vi "Host_Model_Updating.vi"(11 "Setup Parameters and Controls":T3={"Modeling Parameters input controls"={"beam_length"=0.3525, "youngs_modulus"=209500000000.0, "torsion_spring"=0.0, "beam_height"=0.00635, "beam_width"=0.0508, "beam_density"=7900.0, "number_of_FEA_nodes"=40, "accelerometer_mass"=0.055}, "Mockbear input controls"={"Dataset"="test7", "Resample Method"=enum."Auto Resample"}, "Simulation Parameters input controls"={"Eigensolver "=enum."LEMP", "Models Forcasted"=5, "Max Roller Velocity"=3.32, "Max Roller Position Percent"=0.43, "Min Roller Position Percent"=0.155}, "Program Controls"={"Frequency KF"=TRUE, "Pinned State KF"=FALSE, "FFT Bounding"=FALSE, "Filter Constants Frequency"={"Measurement Variance"=0.4, "State Variance"=0.01, "Threshold"=1000000000.0}, "Filter Constants Position"={"Measurement Variance"=0.4, "State Variance"=0.9, "Threshold"=1000000000.0}, "Moving Window Size"=10, "Time Series buffer"=10000.0, "Record Time Series Data"=FALSE, "Record Moving Window Data"=FALSE, "Record Online Error Metrics "=TRUE, "Record Statistics"=TRUE}}) -> ()   [LabVIEW 2021]
uses:
  Model_Updating_Classes/DROPBEAR_Model_Updating/DROPBEAR_Model_Updating.lvclass
panel:
  in  "Halt":bool
  in  "Tab Control":enum32{"Time Series", "Statistics", "Controls"}(tab)
  out "Frequency":dynamicdata(graph)
  out "Meter":dynamicdata(graph)
  out "Nodal":dynamicdata(graph)
  out "DAQ Time cost":T1
  out "FFT Time cost":T1
  out "FEA Time cost":T1
  out "FFT KF Time cost":T1
  out "Sampling Time cost":T1
  out "State KF Time cost":T1
  out "Cycle Time cost":T1
  out "StatisticsTime cost":T1
  out "Signal Quality Stats Frequency":T2
  out "Signal Quality Stats Position":T2
  out "Average Cycle Time (ms)":dbl
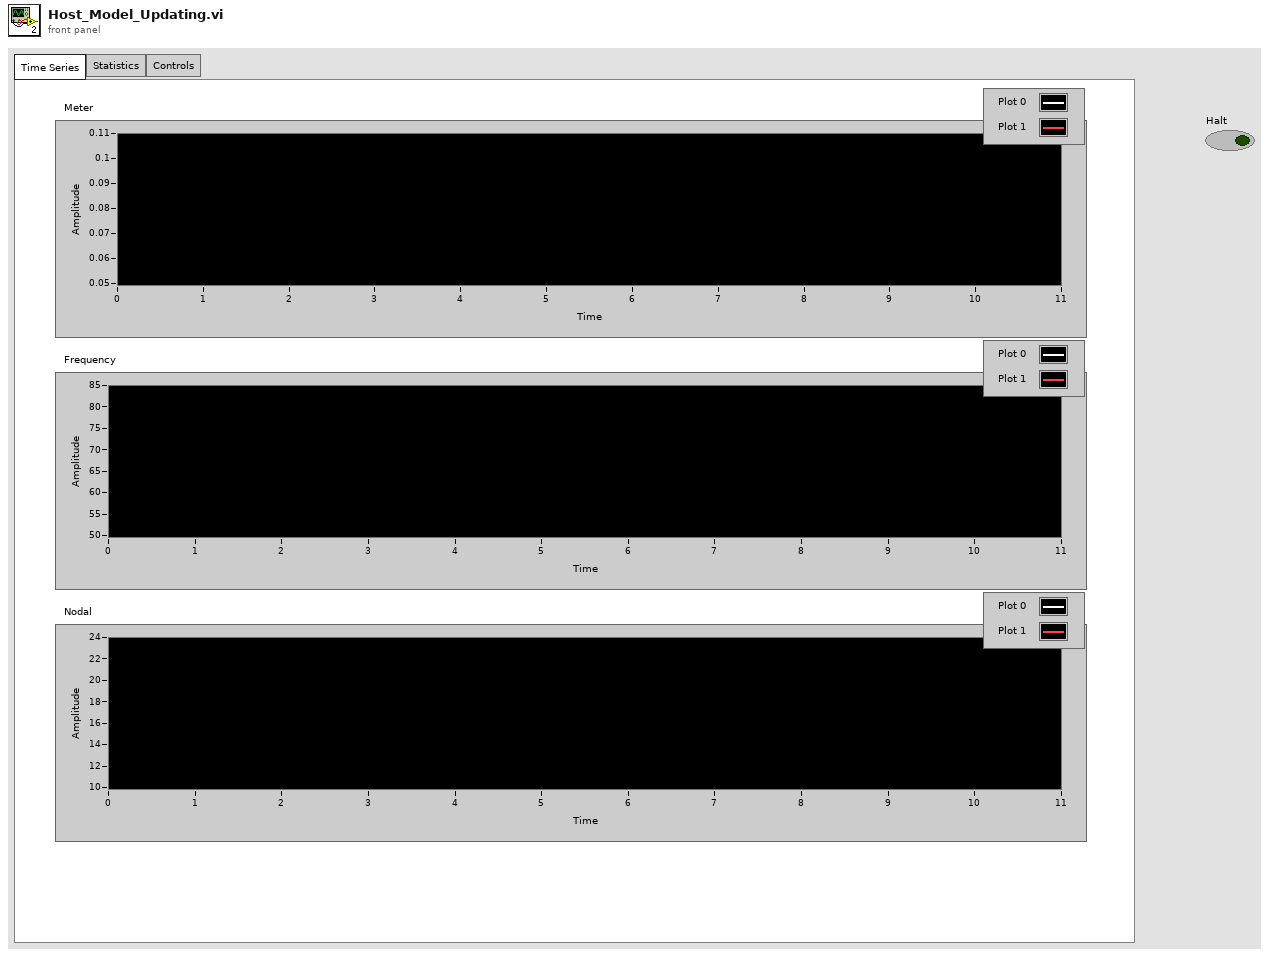
[diagram p1: front panel]
types:
  T1 = cluster{"Cumulative_mean":dbl, "Cumulative_mean_square ":dbl, "Cumulative_variance":dbl, "Max":dbl, "Min":dbl, "Number_of_samples":i32}
  T2 = cluster{"SNR":dbl, "TRAC":dbl, "Cumulative_mean":dbl, "Cumulative_mean_square ":dbl, "Cumulative_variance":dbl, "Max":dbl, "Min":dbl, "Number_of_samples":i32}
  T3 = cluster{"Modeling Parameters input controls":cluster{"beam_length":dbl, "youngs_modulus":dbl, "torsion_spring":dbl, "beam_height":dbl, "beam_width":dbl, "beam_density":dbl, "number_of_FEA_nodes":i32, "accelerometer_mass":dbl}, "Mockbear input controls":cluster{"Dataset":string, "Resample Method":enum16{"Recorded", "Auto Resample", "Custom Resample"}}, "Simulation Parameters input controls":cluster{"Eigensolver ":enum16{"LabVIEW Cholesky", "LabVIEW General", "LabVIEW Inverse", "LEMP"}, "Models Forcasted":i32, "Max Roller Velocity":dbl, "Max Roller Position Percent":dbl, "Min Roller Position Percent":dbl}, "Program Controls":cluster{"Frequency KF":bool, "Pinned State KF":bool, "FFT Bounding":bool, "Filter Constants Frequency":cluster{"Measurement Variance":dbl, "State Variance":dbl, "Threshold":dbl}, "Filter Constants Position":cluster{"Measurement Variance":dbl, "State Variance":dbl, "Threshold":dbl}, "Moving Window Size":i32, "Time Series buffer":dbl, "Record Time Series Data":bool, "Record Moving Window Data":bool, "Record Online Error Metrics ":bool, "Record Statistics":bool}}
  T4 = cluster{"Signal Quality Stats Frequency":cluster{"SNR":dbl, "TRAC":dbl, "Cumulative_mean":dbl, "Cumulative_mean_square ":dbl, "Cumulative_variance":dbl, "Max":dbl, "Min":dbl, "Number_of_samples":i32}, "Signal Quality Stats Position":cluster{"SNR":dbl, "TRAC":dbl, "Cumulative_mean":dbl, "Cumulative_mean_square ":dbl, "Cumulative_variance":dbl, "Max":dbl, "Min":dbl, "Number_of_samples":i32}}
  T5 = cluster{"DAQ Time cost":cluster{"Cumulative_mean":dbl, "Cumulative_mean_square ":dbl, "Cumulative_variance":dbl, "Max":dbl, "Min":dbl, "Number_of_samples":i32}, "FFT Time cost":cluster{"Cumulative_mean":dbl, "Cumulative_mean_square ":dbl, "Cumulative_variance":dbl, "Max":dbl, "Min":dbl, "Number_of_samples":i32}, "FFT KF Time cost":cluster{"Cumulative_mean":dbl, "Cumulative_mean_square ":dbl, "Cumulative_variance":dbl, "Max":dbl, "Min":dbl, "Number_of_samples":i32}, "Sampling Time cost":cluster{"Cumulative_mean":dbl, "Cumulative_mean_square ":dbl, "Cumulative_variance":dbl, "Max":dbl, "Min":dbl, "Number_of_samples":i32}, "FEA Time cost":cluster{"Cumulative_mean":dbl, "Cumulative_mean_square ":dbl, "Cumulative_variance":dbl, "Max":dbl, "Min":dbl, "Number_of_samples":i32}, "State KF Time cost":cluster{"Cumulative_mean":dbl, "Cumulative_mean_square ":dbl, "Cumulative_variance":dbl, "Max":dbl, "Min":dbl, "Number_of_samples":i32}, "Cycle Time cost":cluster{"Cumulative_mean":dbl, "Cumulative_mean_square ":dbl, "Cumulative_variance":dbl, "Max":dbl, "Min":dbl, "Number_of_samples":i32}, "StatisticsTime cost":cluster{"Cumulative_mean":dbl, "Cumulative_mean_square ":dbl, "Cumulative_variance":dbl, "Max":dbl, "Min":dbl, "Number_of_samples":i32}}
  T6 = cluster{"Frequency":dynamicdata, "Meters":dynamicdata, "Nodal":dynamicdata}
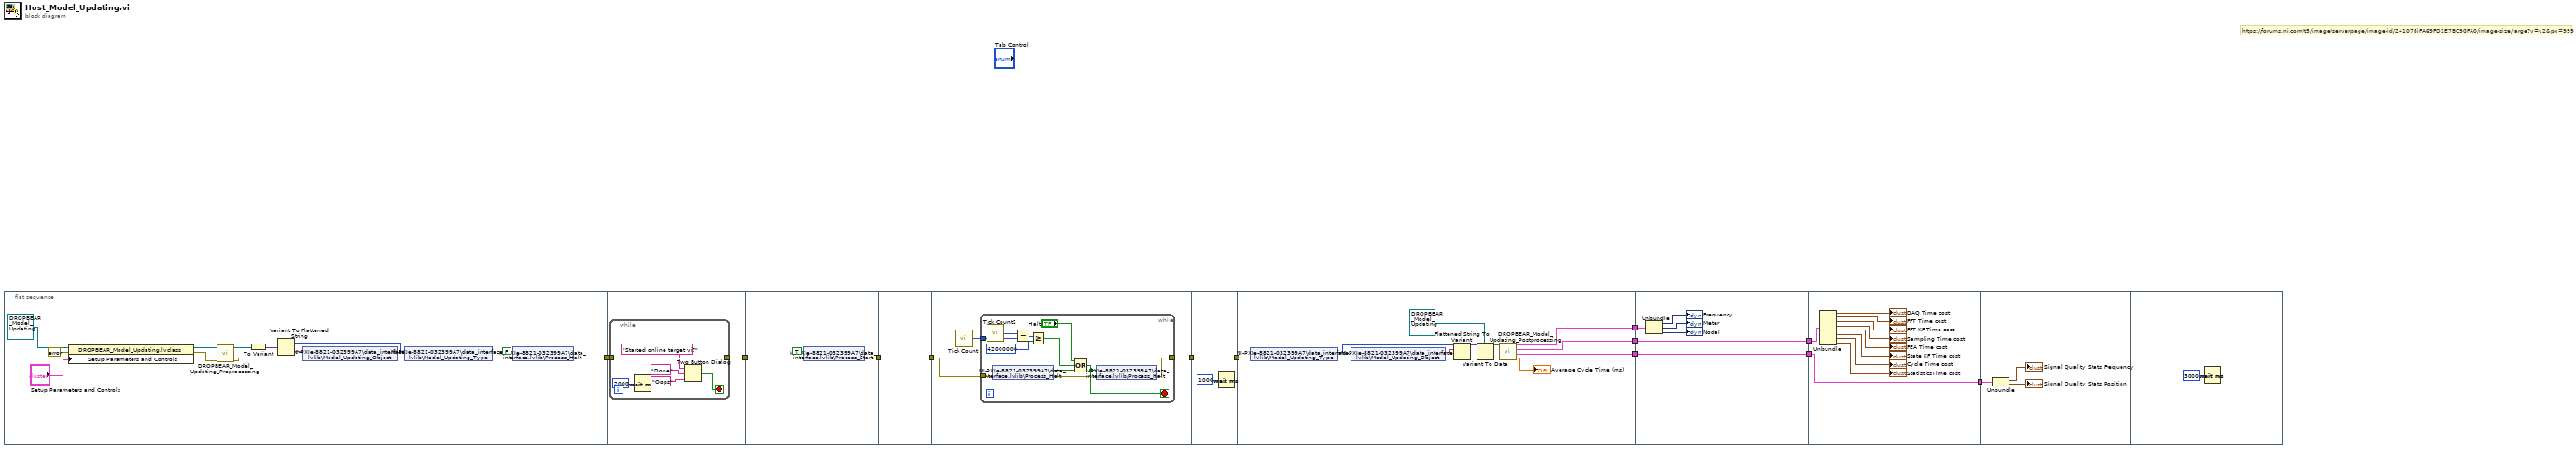
[diagram p0: block diagram]
diagram:
  # "https://forums.ni.com/t5/image/serverpage/image-id/241078iFA69FD1E7BC90FA0/image-size/large?v=v2&px=999"
  n1 = flat-sequence {
    tunnel: [w23] -> w10
    tunnel: w10 -> [w28]
    tunnel: [w27] -> w9
    tunnel: w9 -> [w37]
    tunnel: [w36] -> w12
    tunnel: w12 -> [w38]
    tunnel: [w38] -> w11
    tunnel: w11 -> [w40]
    tunnel: [w39] -> w8
    tunnel: w8 -> [w54]
    tunnel: [w54] -> w7
    tunnel: w7 -> [w60]
    tunnel: [w57] -> w6
    tunnel: [w56] -> w4
    tunnel: [w55] -> w2
    tunnel: w6 -> [w74]
    tunnel: [w73] -> w5
    tunnel: w4 -> [w73]
    tunnel: [w72] -> w3
    tunnel: w2 -> [w72]
    tunnel: w5 -> [w84]
    tunnel: w3 -> [w75]
    tunnel: [w75] -> w1
    tunnel: w1 -> [w87]
    frame #0 {
      n2 = property class="DROPBEAR_Model_Updating.lvclass"(reference=refnum<class "DROPBEAR_Model_Updating.lvclass"> refnum ("DROPBEAR_Model_Updating.lvclass"), error in=errorcluster {"status"=FALSE, "code"=0, "source"=""} ("error in (no error)"), "Setup Parameters and Controls"="Setup Parameters and Controls") -> (reference out=w18:refnum<class "DROPBEAR_Model_Updating.lvclass">, error out=w14:errorcluster)
      n3 = call-dynamic "DROPBEAR_Model_Updating_Preprocessing.vi"("error in (no error)"=w14, "DROPBEAR_Model_Updating in"=w18) -> ("error out"=w25:errorcluster, "DROPBEAR_Model_Updating out"=w26:refnum<class "DROPBEAR_Model_Updating.lvclass">)  [unwired: 8 in]
      n4 = To Variant(anything=w26) -> (Variant=w22:variant)
      n5 = Variant To Flattened String(Variant=w22) -> (data string=w21:string, 1:w13:i16[])
      n6 = shared-variable "NI-PXIe-8821-032399A7\\data_interface.lvlib\\Model_Updating_Object"(w21, error in=w25) -> (error out=w20:errorcluster)
      n7 = shared-variable "NI-PXIe-8821-032399A7\\data_interface.lvlib\\Model_Updating_Type"(w13, error in=w20) -> (error out=w19:errorcluster)
      n8 = shared-variable "NI-PXIe-8821-032399A7\\data_interface.lvlib\\Process_Halt"(FALSE, error in=w19) -> (error out=w23:errorcluster)
    }
    frame #1 {
      n9 = while {
        tunnel: w28 -> [w34]
        tunnel: [w34] -> w27
        stop <- w32 stop-if-true
        n10 = Wait (ms)(milliseconds to wait=u32 2000) -> ()  [unwired: 1 out]
        n11 = Two Button Dialog(message="Started online target vi?", 1:"Oops" ("T button name (\"OK\")"), 2:"Done" ("T button name (\"OK\")")) -> (T button?=w32:bool)
      }
    }
    frame #2 {
      n12 = shared-variable "NI-PXIe-8821-032399A7\\data_interface.lvlib\\Process_Start"(TRUE ("Process_Start"), error in=w37) -> (error out=w36:errorcluster)
    }
    frame #3 {
    }
    frame #4 {
      n13 = call "Tick Count"() -> ("Tick Count(uSec)"=w41:u32)
      n14 = while {
        tunnel: w41 -> [w51]
        tunnel: w40 -> [w45]
        tunnel: [w49] -> w39
        stop <- w48 stop-if-true
        n15 = call "Tick Count2"() -> ("Tick Count(uSec)"=w52:u32)
        n16 = shared-variable "NI-PXIe-8821-032399A7\\data_interface.lvlib\\Process_Halt"(error in=w45) -> (w43:bool, error out=w44:errorcluster)
        n17 = Subtract(x=w52, y=w51) -> (x-y=w42:u32)
        n18 = Greater Or Equal?(x=w42, y=u32 42000000) -> (x >= y?=w46:bool)
        n19 = Compound Arithmetic op=OR("Halt", w46, w43) -> (w48:bool)
        n20 = shared-variable "NI-PXIe-8821-032399A7\\data_interface.lvlib\\Process_Halt"(w48, error in=w44) -> (error out=w49:errorcluster)
      }
    }
    frame #5 {
      n21 = Wait (ms)(milliseconds to wait=u32 1000) -> ()  [unwired: 1 out]
    }
    frame #6 {
      n22 = shared-variable "NI-PXIe-8821-032399A7\\data_interface.lvlib\\Model_Updating_Type"(error in=w60) -> (w64:i16[], error out=w67:errorcluster)
      n23 = shared-variable "NI-PXIe-8821-032399A7\\data_interface.lvlib\\Model_Updating_Object"(error in=w67) -> (w65:string, error out=w66:errorcluster)
      n24 = Flattened String To Variant(4:w66, 6:w65, 7:w64) -> (0:w61:errorcluster, 3:w62:variant)
      n25 = Variant To Data(error in=w61, type=refnum<class "DROPBEAR_Model_Updating.lvclass"> refnum ("DROPBEAR_Model_Updating.lvclass"), Variant=w62) -> (data=w59:refnum<class "DROPBEAR_Model_Updating.lvclass">, error out=w58:errorcluster)
      n26 = call "DROPBEAR_Model_Updating_Postprocessing.vi"("error in (no error)"=w58, "DROPBEAR_Model_Updating in"=w59) -> ("Cycle time (ms)"=→"Average Cycle Time (ms)":dbl, "Signal Quality"=w55:T4, "Timing stats"=w56:T5, "Plots"=w57:T6)  [unwired: 6 in]
    }
    frame #7 {
      n27 = Unbundle(w74) -> ("Frequency"=→"Frequency":dynamicdata, "Meters"=→"Meter":dynamicdata, "Nodal"=→"Nodal":dynamicdata)
    }
    frame #8 {
      n28 = Unbundle(w84) -> ("DAQ Time cost"=→"DAQ Time cost":T1, "FFT Time cost"=→"FFT Time cost":T1, "FFT KF Time cost"=→"FFT KF Time cost":T1, "Sampling Time cost"=→"Sampling Time cost":T1, "FEA Time cost"=→"FEA Time cost":T1, "State KF Time cost"=→"State KF Time cost":T1, "Cycle Time cost"=→"Cycle Time cost":T1, "StatisticsTime cost"=→"StatisticsTime cost":T1)
    }
    frame #9 {
      n29 = Unbundle(w87) -> ("Signal Quality Stats Frequency"=→"Signal Quality Stats Frequency":T2, "Signal Quality Stats Position"=→"Signal Quality Stats Position":T2)
    }
    frame #10 {
      n30 = Wait (ms)(milliseconds to wait=u32 3000) -> ()  [unwired: 1 out]
    }
  }
